vi "ConvertPrefStrings.vi"(6 "Comma?":bool, 8 "String In":string, 11 "Settings":T1={"Name of test"="", "Date"=timestamp(0 s since 1904-01-01), "Location"="Home", "Template"="Simple", "Soundcard"="OCTA-CAPTURE", "resolution"=32, "Sampling rate"=48000, "Ch1 Gain "=25.0, "Ch2 Gain"=10.0, "Sample time (s)"=0.3, "Pre-trigger (s)"=0.001, "Hammer Threshold"=10.0, "Positions"=12, "Taps/Position"=5, "Set Names"="H,V", "Freq resolution"=1.0, "Hammer cutoff"=0.025, "Mic cutoff"=0.25, "Double bounce "=10.0, "Hammer Cal"=10.0, "dB Offset"=0.0, "Accel Cal"=10.0, "Vibrometer Cal"=0.0, "Mic Cal"=0.0, "Output"=2, "Voltage Cal"=0.01, "Vibrometer Port"="ASRL27::INSTR", "Range"=4, "High Pass"=2, "Bandwidth"=4, "X Range"=[], "Y Range"=[], "dB Spread"=0.0, "Trigger"=0, "Ch_1"=25, "Ch_2"=25, "flip?"=FALSE, "60Hz"=FALSE, "Time offset"=0.0, "Piezo Cal"=1.0, "Default Notes"="", "Tom"=FALSE} {"Ch_2" min=1 step=1; "Ch_1" min=1 max=100 step=1; "Trigger" items=["Hammer (force)", "Self-tap", "Spacebar"]; "Bandwidth" items=["1 kHz"=1, "5 kHz"=5, "10 kHz"=10, "25 kHz"=25, "50 kHz"=50, "100 kHz"=100]; "High Pass" items=["Off", "13 Hz", "104 Hz"]; "Range" items=["10 mm/s"=1, "20 mm/s"=2, "50 mm/s"=5, "100 mm/s"=10, "200 mm/s"=20, "500 mm/s"=50, "1 m/s"=100, "2 m/s"=200]; "Output" items=["Accelerometer", "Speed (from acceleration)", "Microphone", "Vibrometer", "Piezo"]; "Voltage Cal" format="%#_13g"; "Ch2 Gain" format="%#_13g"; "Ch1 Gain" format="%#_13g"; "Double bounce" min=0.0; "Mic cutoff" min=0.0 format="%#_4g"; "Hammer cutoff" min=0.0 format="%#_4g"; "Freq resolution" min=0.0; "Pre-trigger (s)" format="%#_13g"; "Date" format="%<%H:%M\n%d/%m/%y>T"; "resolution" items=["16 bit"=16, "24 bit"=24, "32 bit"=32]; "Sampling rate" items=["22050 samp/s"=22050, "44100 samp/s"=44100, "48000 samp/s"=48000]}) -> (0 "Settings":T1={"Name of test"="", "Date"=timestamp(0 s since 1904-01-01), "Location"="", "Template"="", "Soundcard"="", "resolution"=32, "Sampling rate"=48000, "Ch1 Gain "=25.0, "Ch2 Gain"=10.0, "Sample time (s)"=0.3, "Pre-trigger (s)"=0.01, "Hammer Threshold"=10.0, "Positions"=12, "Taps/Position"=5, "Set Names"="", "Freq resolution"=10.0, "Hammer cutoff"=0.0, "Mic cutoff"=0.0, "Double bounce "=0.0, "Hammer Cal"=10.0, "dB Offset"=0.0, "Accel Cal"=10.0, "Vibrometer Cal"=0.0, "Mic Cal"=0.0, "Output"=2, "Voltage Cal"=0.01, "Vibrometer Port"="ASRL27::INSTR", "Range"=4, "High Pass"=2, "Bandwidth"=4, "X Range"=[], "Y Range"=[], "dB Spread"=0.0, "Trigger"=0, "Ch_1"=25, "Ch_2"=25, "flip?"=FALSE, "60Hz"=FALSE, "Time offset"=0.0, "Piezo Cal"=1.0, "Default Notes"="", "Tom"=FALSE} {"Ch_2" min=1 step=1; "Ch_1" min=1 max=100 step=1; "Trigger" items=["Hammer (force)", "Self-tap", "Spacebar"]; "Bandwidth" items=["1 kHz"=1, "5 kHz"=5, "10 kHz"=10, "25 kHz"=25, "50 kHz"=50, "100 kHz"=100]; "High Pass" items=["Off", "13 Hz", "104 Hz"]; "Range" items=["10 mm/s"=1, "20 mm/s"=2, "50 mm/s"=5, "100 mm/s"=10, "200 mm/s"=20, "500 mm/s"=50, "1 m/s"=100, "2 m/s"=200]; "Output" items=["Accelerometer", "Speed (from acceleration)", "Microphone", "Vibrometer", "Piezo"]; "Voltage Cal" format="%#_13g"; "Ch2 Gain" format="%#_13g"; "Ch1 Gain" format="%#_13g"; "Double bounce" min=0.0; "Mic cutoff" min=0.0 format="%#_4g"; "Hammer cutoff" min=0.0 format="%#_4g"; "Freq resolution" min=0.0; "Pre-trigger (s)" format="%#_13g"; "Date" format="%<%H:%M\n%d/%m/%y>T"; "resolution" items=["16 bit"=16, "24 bit"=24, "32 bit"=32]; "Sampling rate" items=["22050 samp/s"=22050, "44100 samp/s"=44100, "48000 samp/s"=48000]}, 3 "String Out":string)   [LabVIEW 2022 SP3]
uses:
  Mic/Mic_Global.vi
  PreferencesControl.ctl
panel:
  # "Hz"
  # "dB"
  # "dB"
  # "sec"
  # "sec"
  # "mV/Pa"
  # "mV/m/s2"
  # "mV/mm/s"
  # "V/N"
  # "sec"
  # "sec"
  # "mV/N"
  # "%"
  # "%"
  # "sec"
  # "Hz"
  # "dB"
  # "dB"
  # "sec"
  # "sec"
  # "mV/Pa"
  # "mV/m/s2"
  # "mV/mm/s"
  # "V/N"
  # "sec"
  # "sec"
  # "mV/N"
  # "%"
  # "%"
  # "sec"
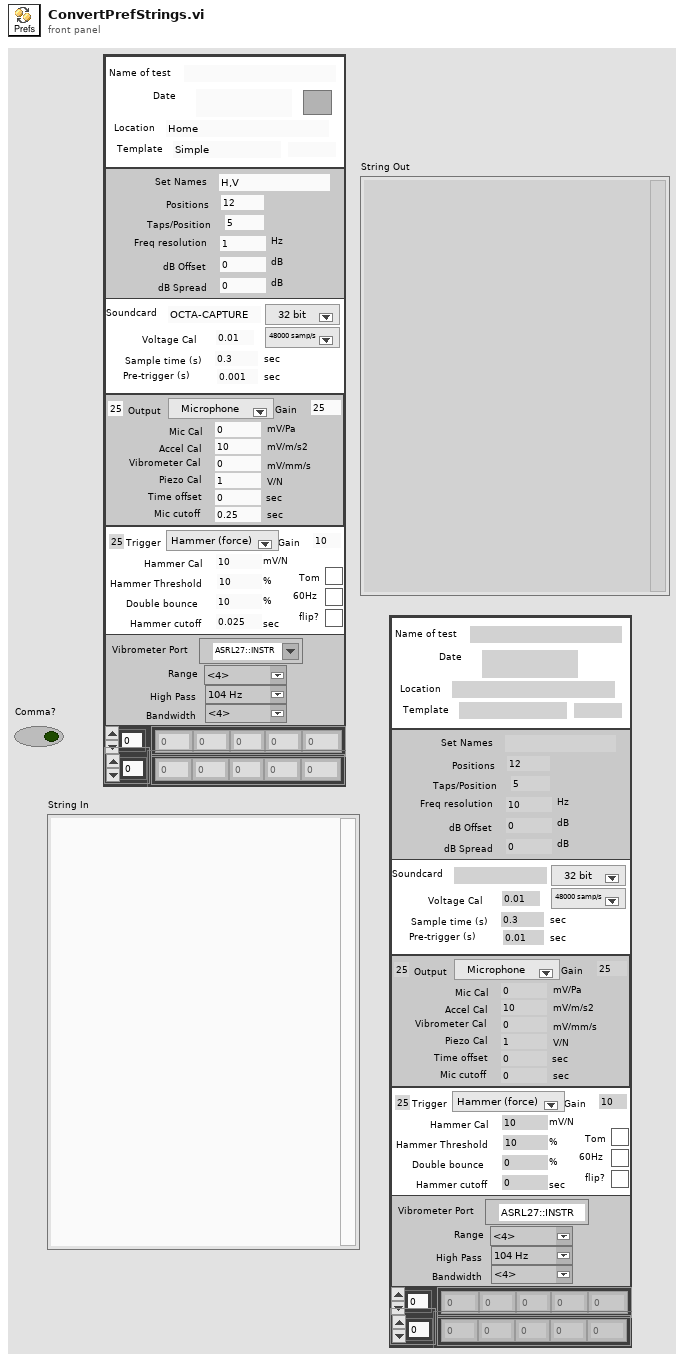
[diagram p1: front panel]
types:
  T1 = typedef "PreferencesControl.ctl" = cluster{"Name of test":string, "Date":timestamp, "Location":string, "Template":string, "Soundcard":string, "resolution":u16, "Sampling rate":u16, "Ch1 Gain ":dbl, "Ch2 Gain":dbl, "Sample time (s)":dbl, "Pre-trigger (s)":dbl, "Hammer Threshold":dbl, "Positions":i16, "Taps/Position":i16, "Set Names":string, "Freq resolution":dbl, "Hammer cutoff":dbl, "Mic cutoff":dbl, "Double bounce ":dbl, "Hammer Cal":dbl, "dB Offset":dbl, "Accel Cal":dbl, "Vibrometer Cal":dbl, "Mic Cal":dbl, "Output":u16, "Voltage Cal":dbl, "Vibrometer Port":refnum<visa-resource-name>, "Range":u16, "High Pass":u16, "Bandwidth":u16, "X Range":cluster{"Minimum":dbl, "Maximum":dbl, "Increment":dbl, "Minor Increment":dbl, "Start":dbl}[], "Y Range":cluster{"Minimum":dbl, "Maximum":dbl, "Increment":dbl, "Minor Increment":dbl, "Start":dbl}[], "dB Spread":dbl, "Trigger":u16, "Ch_1":u8, "Ch_2":u8, "flip?":bool, "60Hz":bool, "Time offset":dbl, "Piezo Cal":dbl, "Default Notes":string, "Tom":bool}
  T2 = typedef "LVStringsAndValuesArrayTypeDef_U16.ctl" = cluster{"String":string, "Value":u16}[]
  T3 = cluster{"Minimum":dbl, "Maximum":dbl, "Increment":dbl, "Minor Increment":dbl, "Start":dbl}[]
  T4 = cluster{"[0]":dbl, "[1]":dbl, "[2]":dbl, "[3]":dbl, "[4]":dbl}
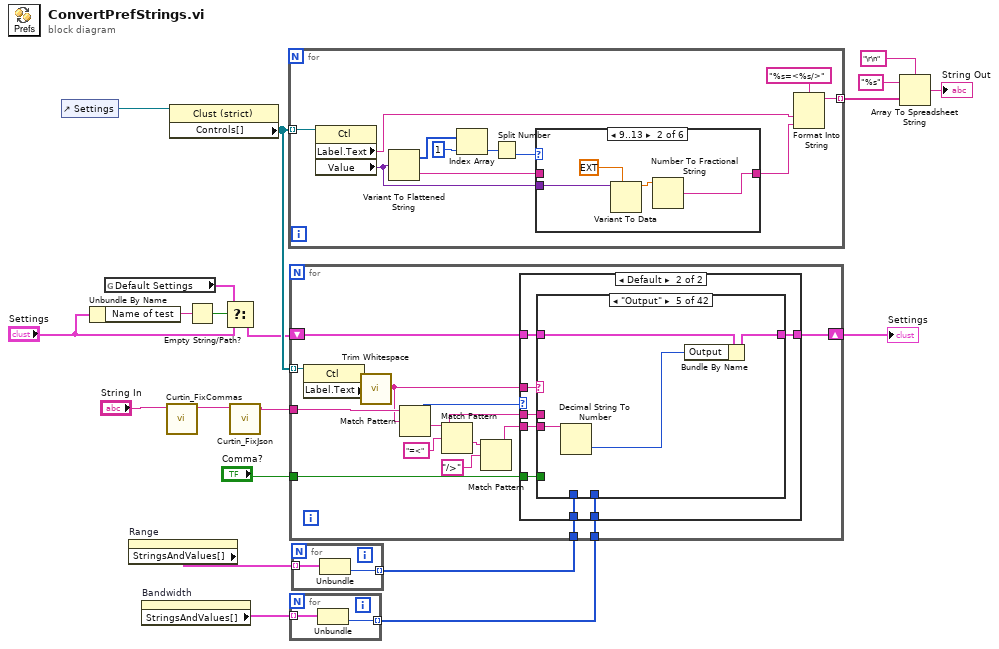
[diagram p0: block diagram]
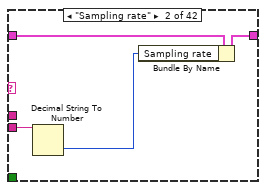
[diagram p4: hidden frame]
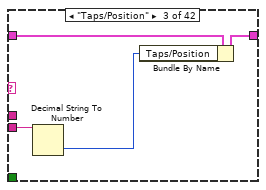
[diagram p5: hidden frame]
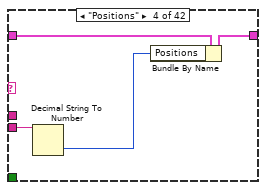
[diagram p6: hidden frame]
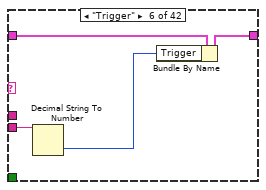
[diagram p7: hidden frame]
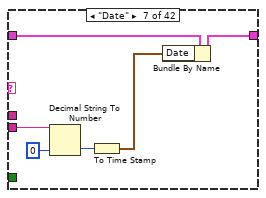
[diagram p8: hidden frame]
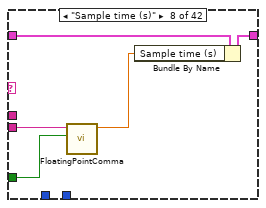
[diagram p9: hidden frame]
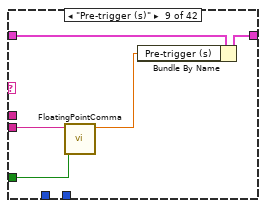
[diagram p10: hidden frame]
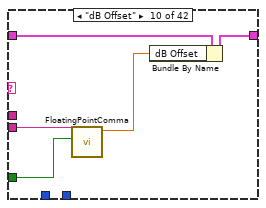
[diagram p11: hidden frame]
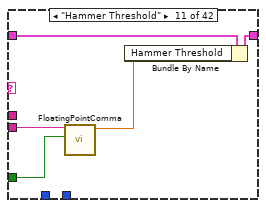
[diagram p12: hidden frame]
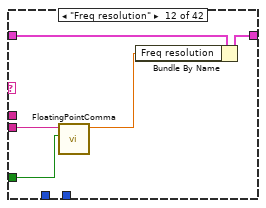
[diagram p13: hidden frame]
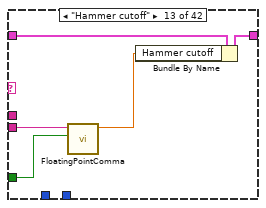
[diagram p14: hidden frame]
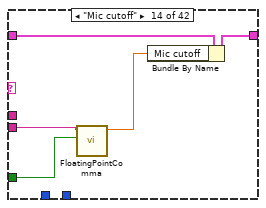
[diagram p15: hidden frame]
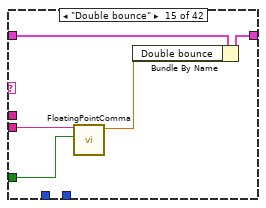
[diagram p16: hidden frame]
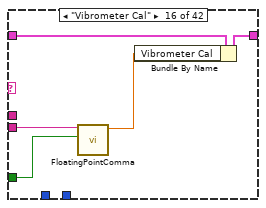
[diagram p17: hidden frame]
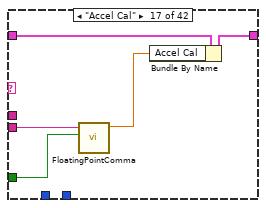
[diagram p18: hidden frame]
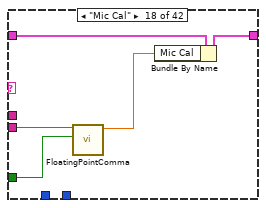
[diagram p19: hidden frame]
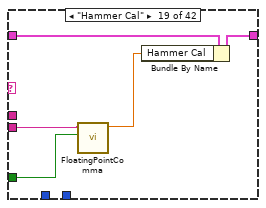
[diagram p20: hidden frame]
diagram:
  n1 = control-ref of="Settings"() -> (w14:refnum<vi>)
  n2 = Unbundle By Name("Settings") -> ("Name of test"=w13:string)
  n3 = global read "Mic_Global.vi" "Default Settings"() -> (w9:T1)
  n4 = property on="Range" class="Ring (strict)"() -> ("StringsAndValues[]"=w7:T2)  [unwired: 2 in, 2 out]
  n5 = property on="Bandwidth" class="Ring (strict)"() -> ("StringsAndValues[]"=w4:T2)  [unwired: 2 in, 2 out]
  n6 = call "Curtin_FixCommas.vi"("String In"="String In") -> ("String In 2"=w2:string)  [unwired: 10 in]
  n7 = property class="Clust (strict)"(reference=w14) -> ("Controls[]"=w16:refnum<vi>[])  [unwired: 1 in, 2 out]
  n8 = Empty String/Path?(string/path=w13) -> (empty?=w12:bool)
  n9 = Select(t=w9, s=w12, f="Settings") -> (s? t:f=w10:T1)
  n10 = call "Curtin_FixJson.vi"("String In"=w2) -> ("String out"=w1:string)  [unwired: 10 in]
  n11 = for {
    tunnel: w16 -> [w31] mode=indexing
    tunnel: [w29] -> w20 mode=indexing
    n12 = property class="Ctl"(reference=w31) -> ("Label.Text"=w22:string, "Value"=w23:variant)  [unwired: 1 in, 2 out]
    n13 = Variant To Flattened String(Variant=w23) -> (data string=w24:string, 1:w28:i16[])
    n14 = Index Array(array=w28, index=1) -> (element=w27:i16)
    n15 = Split Number(x=w27) -> (lo(x)=w21:u8)  [unwired: 1 out]
    n16 = case shown="9..13" w21 {
      tunnel: w23 -> [w35 w39 w45 w50 w56 _]
      tunnel: [w32 w36 w41 w46 w52 w63] -> w25
      tunnel: w24 -> [_ _ _ _ _ w66]
      frame 1..8 {
        n17 = Variant To Data(type=i64 0, Variant=w35) -> (data=w33:i64)  [unwired: 1 in, 1 out]
        n18 = Number To Decimal String(number=w33) -> (decimal integer string=w32:string)  [unwired: 1 in]
      }
      frame 9..13 {
        n19 = Variant To Data(type=ext 0.0, Variant=w39) -> (data=w37:ext)  [unwired: 1 in, 1 out]
        n20 = Number To Fractional String(number=w37) -> (F-format string=w36:string)  [unwired: 3 in]
      }
      frame 31, 33 {
        n21 = Variant To Data(type=FALSE, Variant=w45) -> (data=w43:bool)  [unwired: 1 in, 1 out]
        n22 = Select(t="true", s=w43, f="false") -> (s? t:f=w41:string)
      }
      frame 84 {
        n23 = Variant To Data(type=timestamp(0 s since 1904-01-01), Variant=w50) -> (data=w48:timestamp)  [unwired: 1 in, 1 out]
        n24 = To Unsigned Quad Integer(1:w48) -> (0:w47:u64)
        n25 = Number To Decimal String(number=w47) -> (decimal integer string=w46:string)  [unwired: 1 in]
      }
      frame 64 {
        n26 = Variant To Data(type=T3 [] ("X Range"), Variant=w56) -> (data=w54:T3)  [unwired: 1 in, 1 out]
        n27 = for {
          tunnel: w54 -> [w58] mode=indexing
          tunnel: [w57] -> w53 mode=indexing
          n28 = Cluster To Array(cluster=w58) -> (array=w57:dbl[])
        }
        n29 = Array To Spreadsheet String(array=w53, 3:"%e" ("format string")) -> (spreadsheet string=w52:string)  [unwired: 1 in]
      }
      frame 46, Default {
        n30 = Search/Split String(string=w66, offset (0)=4) -> (substring before match=w61:string, match + rest of string=w64:string)  [unwired: 1 in, 1 out]
        n31 = String To Byte Array(string=w61) -> (unsigned byte array=w60:u8[])
        n32 = Type Cast(type=4 ("offset (0)"), x=w60) -> ()  [unwired: 1 out]
        n33 = Format Into String(format string="%s", w64) -> (resulting string=w63:string)  [unwired: 2 in, 1 out]
      }
    }
    n34 = Format Into String(format string="%s=<%s/>", w22, w25) -> (resulting string=w29:string)  [unwired: 2 in, 1 out]
  }
  n35 = for {
    tunnel: w4 -> [w68] mode=indexing
    tunnel: [w67] -> w5 mode=indexing
    n36 = Unbundle(w68) -> ("Value"=w67:u16)  [unwired: 1 out]
  }
  n37 = for {
    tunnel: w7 -> [w70] mode=indexing
    tunnel: [w69] -> w6 mode=indexing
    n38 = Unbundle(w70) -> ("Value"=w69:u16)  [unwired: 1 out]
  }
  n39 = for {
    tunnel: w1 -> [w76]
    tunnel: w16 -> [w82] mode=indexing
    shift-right: [w80] -> w15
    shift-left: w10 -> [w81]
    tunnel: w6 -> [w73]
    tunnel: w5 -> [w72]
    tunnel: "Comma?" -> [w71]
    n40 = property class="Ctl"(reference=w82) -> ("Label.Text"=w75:string)  [unwired: 1 in, 2 out]
    n41 = call <vilib>:"Trim Whitespace.vi"("string"=w75) -> ("trimmed string"=w74:string)  [unwired: 1 in]
    n42 = Match Pattern(string=w76, regular expression=w74) -> (after substring=w77:string, offset past match=w78:i32)  [unwired: 1 in, 2 out]
    n43 = Match Pattern(string=w77, regular expression="=<" ("format string")) -> (after substring=w83:string)  [unwired: 1 in, 3 out]
    n44 = Match Pattern(string=w83, regular expression="/>" ("format string")) -> (before substring=w79:string)  [unwired: 1 in, 3 out]
    n45 = case shown="Default" w78 {
      tunnel: w81 -> [w86 w94]
      tunnel: [w86 w93] -> w80
      tunnel: w74 -> [_ w92]
      tunnel: w79 -> [_ w91]
      tunnel: w77 -> [_ w90]
      tunnel: w73 -> [_ w89]
      tunnel: w72 -> [_ w88]
      tunnel: w71 -> [_ w87]
      frame -1 {
      }
      frame Default {
        n46 = case shown="\"Output\"" w92 {
          tunnel: w94 -> [w95 w99 w103 w107 w111 w115 w121 w126 w131 w136 w141 w146 w151 w156 w161 w166 w171 w176 w181 w185 w188 w191 w194 w197 w200 w205 w210 w215 w218 w221 w230 w234 w243 w251 w261 w268 w272 w276 w281 w286 w291 w296]
          tunnel: [w95 w98 w102 w106 w110 w114 w120 w125 w130 w135 w140 w145 w150 w155 w160 w165 w170 w175 w180 w184 w187 w190 w193 w196 w199 w204 w209 w214 w217 w220 w229 w233 w242 w250 w260 w267 w271 w275 w280 w285 w290 w295] -> w93
          tunnel: w91 -> [_ w97 w101 w105 w109 w113 w119 w124 w129 w134 w139 w144 w149 w154 w159 w164 w169 w174 w179 w183 w186 w189 w192 w195 w198 w203 w208 w212 w216 w219 w223 w232 w241 w246 w256 w266 w270 w274 w278 w283 w288 w294]
          tunnel: w90 -> [_ _ _ _ _ _ _ _ _ _ _ _ _ _ _ _ _ _ _ _ _ _ _ _ _ _ _ _ _ _ _ _ _ _ _ _ _ _ _ _ _ _]
          tunnel: w89 -> [_ _ _ _ _ _ _ _ _ _ _ _ _ _ _ _ _ _ _ _ _ _ _ _ _ _ _ _ _ _ w222 _ _ _ _ _ _ _ _ _ _ _]
          tunnel: w88 -> [_ _ _ _ _ _ _ _ _ _ _ _ _ _ _ _ _ _ _ _ _ _ _ _ _ _ _ _ _ _ _ _ w237 _ _ _ _ _ _ _ _ _]
          tunnel: w87 -> [_ _ _ _ _ _ _ w122 w128 w133 w138 w143 w148 w153 w158 w163 w168 w173 w178 _ _ _ _ _ _ w202 w207 w213 _ _ _ _ _ w245 w255 w265 _ _ _ _ _ w293]
          frame Default {
          }
          frame "Sampling rate" {
            n47 = Decimal String To Number(string=w97) -> (number=w96:i32)  [unwired: 2 in, 1 out]
            n48 = Bundle By Name(cluster=w99, "Sampling rate"=w96) -> (w98:T1)
          }
          frame "Taps/Position" {
            n49 = Decimal String To Number(string=w101) -> (number=w100:i32)  [unwired: 2 in, 1 out]
            n50 = Bundle By Name(cluster=w103, "Taps/Position"=w100) -> (w102:T1)
          }
          frame "Positions" {
            n51 = Decimal String To Number(string=w105) -> (number=w104:i32)  [unwired: 2 in, 1 out]
            n52 = Bundle By Name(cluster=w107, "Positions"=w104) -> (w106:T1)
          }
          frame "Output" {
            n53 = Decimal String To Number(string=w109) -> (number=w108:i32)  [unwired: 2 in, 1 out]
            n54 = Bundle By Name(cluster=w111, "Output"=w108) -> (w110:T1)
          }
          frame "Trigger" {
            n55 = Decimal String To Number(string=w113) -> (number=w112:i32)  [unwired: 2 in, 1 out]
            n56 = Bundle By Name(cluster=w115, "Trigger"=w112) -> (w114:T1)
          }
          frame "Date" {
            n57 = Decimal String To Number(string=w119, default (0L)=u64 0 ("default (0 I32)")) -> (number=w118:u64)  [unwired: 1 in, 1 out]
            n58 = To Time Stamp(1:w118) -> (0:w117:timestamp)
            n59 = Bundle By Name(cluster=w121, "Date"=w117) -> (w120:T1)
          }
          frame "Sample time (s)" {
            n60 = call "FloatingPointComma.vi"("Comma?"=w122, "String In"=w124) -> ("Numeric"=w123:dbl)  [unwired: 8 in, 1 out]
            n61 = Bundle By Name(cluster=w126, "Sample time (s)"=w123) -> (w125:T1)
          }
          frame "Pre-trigger (s)" {
            n62 = call "FloatingPointComma.vi"("Comma?"=w128, "String In"=w129) -> ("Numeric"=w127:dbl)  [unwired: 8 in, 1 out]
            n63 = Bundle By Name(cluster=w131, "Pre-trigger (s)"=w127) -> (w130:T1)
          }
          frame "dB Offset" {
            n64 = call "FloatingPointComma.vi"("Comma?"=w133, "String In"=w134) -> ("Numeric"=w132:dbl)  [unwired: 8 in, 1 out]
            n65 = Bundle By Name(cluster=w136, "dB Offset"=w132) -> (w135:T1)
          }
          frame "Hammer Threshold" {
            n66 = call "FloatingPointComma.vi"("Comma?"=w138, "String In"=w139) -> ("Numeric"=w137:dbl)  [unwired: 8 in, 1 out]
            n67 = Bundle By Name(cluster=w141, "Hammer Threshold"=w137) -> (w140:T1)
          }
          frame "Freq resolution" {
            n68 = call "FloatingPointComma.vi"("Comma?"=w143, "String In"=w144) -> ("Numeric"=w142:dbl)  [unwired: 8 in, 1 out]
            n69 = Bundle By Name(cluster=w146, "Freq resolution"=w142) -> (w145:T1)
          }
          frame "Hammer cutoff" {
            n70 = call "FloatingPointComma.vi"("Comma?"=w148, "String In"=w149) -> ("Numeric"=w147:dbl)  [unwired: 8 in, 1 out]
            n71 = Bundle By Name(cluster=w151, "Hammer cutoff"=w147) -> (w150:T1)
          }
          frame "Mic cutoff" {
            n72 = call "FloatingPointComma.vi"("Comma?"=w153, "String In"=w154) -> ("Numeric"=w152:dbl)  [unwired: 8 in, 1 out]
            n73 = Bundle By Name(cluster=w156, "Mic cutoff"=w152) -> (w155:T1)
          }
          frame "Double bounce" {
            n74 = call "FloatingPointComma.vi"("Comma?"=w158, "String In"=w159) -> ("Numeric"=w157:dbl)  [unwired: 8 in, 1 out]
            n75 = Bundle By Name(cluster=w161, "Double bounce"=w157) -> (w160:T1)
          }
          frame "Vibrometer Cal" {
            n76 = call "FloatingPointComma.vi"("Comma?"=w163, "String In"=w164) -> ("Numeric"=w162:dbl)  [unwired: 8 in, 1 out]
            n77 = Bundle By Name(cluster=w166, "Vibrometer Cal"=w162) -> (w165:T1)
          }
          frame "Accel Cal" {
            n78 = call "FloatingPointComma.vi"("Comma?"=w168, "String In"=w169) -> ("Numeric"=w167:dbl)  [unwired: 8 in, 1 out]
            n79 = Bundle By Name(cluster=w171, "Accel Cal"=w167) -> (w170:T1)
          }
          frame "Mic Cal" {
            n80 = call "FloatingPointComma.vi"("Comma?"=w173, "String In"=w174) -> ("Numeric"=w172:dbl)  [unwired: 8 in, 1 out]
            n81 = Bundle By Name(cluster=w176, "Mic Cal"=w172) -> (w175:T1)
          }
          frame "Hammer Cal" {
            n82 = call "FloatingPointComma.vi"("Comma?"=w178, "String In"=w179) -> ("Numeric"=w177:dbl)  [unwired: 8 in, 1 out]
            n83 = Bundle By Name(cluster=w181, "Hammer Cal"=w177) -> (w180:T1)
          }
          frame "resolution" {
            n84 = Decimal String To Number(string=w183) -> (number=w182:i32)  [unwired: 2 in, 1 out]
            n85 = Bundle By Name(cluster=w185, "resolution"=w182) -> (w184:T1)
          }
          frame "Soundcard" {
            n86 = Bundle By Name(cluster=w188, "Soundcard"=w186) -> (w187:T1)
          }
          frame "Name of test" {
            n87 = Bundle By Name(cluster=w191, "Name of test"=w189) -> (w190:T1)
          }
          frame "Set Names" {
            n88 = Bundle By Name(cluster=w194, "Set Names"=w192) -> (w193:T1)
          }
          frame "Location" {
            n89 = Bundle By Name(cluster=w197, "Location"=w195) -> (w196:T1)
          }
          frame "Default Template" {
            n90 = Bundle By Name(cluster=w200, "Template"=w198) -> (w199:T1)
          }
          frame "Ch1 Gain" {
            n91 = call "FloatingPointComma.vi"("Comma?"=w202, "String In"=w203) -> ("Numeric"=w201:dbl)  [unwired: 8 in, 1 out]
            n92 = Bundle By Name(cluster=w205, "Ch1 Gain"=w201) -> (w204:T1)
          }
          frame "Ch2 Gain" {
            n93 = call "FloatingPointComma.vi"("Comma?"=w207, "String In"=w208) -> ("Numeric"=w206:dbl)  [unwired: 8 in, 1 out]
            n94 = Bundle By Name(cluster=w210, "Ch2 Gain"=w206) -> (w209:T1)
          }
          frame "Voltage Cal" {
            n95 = call "FloatingPointComma.vi"("Comma?"=w213, "String In"=w212) -> ("Numeric"=w211:dbl)  [unwired: 8 in, 1 out]
            n96 = Bundle By Name(cluster=w215, "Voltage Cal"=w211) -> (w214:T1)
          }
          frame "Vibrometer Port" {
            n97 = Bundle By Name(cluster=w218, "Vibrometer Port"=w216) -> (w217:T1)
          }
          frame "Default Notes" {
            n98 = Bundle By Name(cluster=w221, "Default Notes"=w219) -> (w220:T1)
          }
          frame "Range" {
            n99 = Decimal String To Number(string=w223) -> (number=w226:i32)  [unwired: 2 in, 1 out]
            n100 = Search 1D Array(1D array=w222, element=w226) -> (index of element=w228:i32)  [unwired: 1 in]
            n101 = Greater Or Equal To 0?(x=w228) -> (x >= 0?=w227:bool)
            n102 = Select(t=w226, s=w227, f=20) -> (s? t:f=w225:i32)
            n103 = Bundle By Name(cluster=w230, "Range"=w225) -> (w229:T1)
          }
          frame "High Pass" {
            n104 = Decimal String To Number(string=w232) -> (number=w231:i32)  [unwired: 2 in, 1 out]
            n105 = Bundle By Name(cluster=w234, "High Pass"=w231) -> (w233:T1)
          }
          frame "Bandwidth" {
            n106 = Decimal String To Number(string=w241) -> (number=w236:i32)  [unwired: 2 in, 1 out]
            n107 = Search 1D Array(1D array=w237, element=w236) -> (index of element=w240:i32)  [unwired: 1 in]
            n108 = Greater Or Equal To 0?(x=w240) -> (x >= 0?=w239:bool)
            n109 = Select(t=w236, s=w239, f=25) -> (s? t:f=w235:i32)
            n110 = Bundle By Name(cluster=w243, "Bandwidth"=w235) -> (w242:T1)
          }
          frame "X Range" {
            n111 = call "FloatingPointComma.vi"("Comma?"=w245, "String In"=w246) -> ("fixed"=w244:string)  [unwired: 8 in, 1 out]
            n112 = Spreadsheet String To Array(format string="%e", spreadsheet string=w244) -> (array=w248:dbl[][])  [unwired: 2 in]
            n113 = for {
              tunnel: w248 -> [w253] mode=indexing
              tunnel: [w252] -> w247 mode=indexing
              n114 = Array To Cluster(array=w253) -> (cluster=w252:T4)
            }
            n115 = Bundle By Name(cluster=w251, "X Range"=w247) -> (w250:T1)
          }
          frame "Y Range" {
            n116 = call "FloatingPointComma.vi"("Comma?"=w255, "String In"=w256) -> ("fixed"=w254:string)  [unwired: 8 in, 1 out]
            n117 = Spreadsheet String To Array(format string="%e", spreadsheet string=w254) -> (array=w258:dbl[][])  [unwired: 2 in]
            n118 = for {
              tunnel: w258 -> [w263] mode=indexing
              tunnel: [w262] -> w257 mode=indexing
              n119 = Array To Cluster(array=w263) -> (cluster=w262:T4)
            }
            n120 = Bundle By Name(cluster=w261, "Y Range"=w257) -> (w260:T1)
          }
          frame "dB Spread" {
            n121 = call "FloatingPointComma.vi"("Comma?"=w265, "String In"=w266) -> ("Numeric"=w264:dbl)  [unwired: 8 in, 1 out]
            n122 = Bundle By Name(cluster=w268, "dB Spread"=w264) -> (w267:T1)
          }
          frame "Ch_1" {
            n123 = Decimal String To Number(string=w270) -> (number=w269:i32)  [unwired: 2 in, 1 out]
            n124 = Bundle By Name(cluster=w272, "Ch_1"=w269) -> (w271:T1)
          }
          frame "Ch_2" {
            n125 = Decimal String To Number(string=w274) -> (number=w273:i32)  [unwired: 2 in, 1 out]
            n126 = Bundle By Name(cluster=w276, "Ch_2"=w273) -> (w275:T1)
          }
          frame "flip?" {
            n127 = Equal?(x="true", y=w278) -> (x = y?=w277:bool)
            n128 = Bundle By Name(cluster=w281, "flip?"=w277) -> (w280:T1)
          }
          frame "60Hz" {
            n129 = Equal?(x="true", y=w283) -> (x = y?=w282:bool)
            n130 = Bundle By Name(cluster=w286, "60Hz"=w282) -> (w285:T1)
          }
          frame "Tom" {
            n131 = Equal?(x="true", y=w288) -> (x = y?=w287:bool)
            n132 = Bundle By Name(cluster=w291, "Tom"=w287) -> (w290:T1)
          }
          frame "Time offset" {
            n133 = call "FloatingPointComma.vi"("Comma?"=w293, "String In"=w294) -> ("Numeric"=w292:dbl)  [unwired: 8 in, 1 out]
            n134 = Bundle By Name(cluster=w296, "Time offset"=w292) -> (w295:T1)
          }
        }
      }
    }
  }
  "Settings" <- w15
  n135 = Array To Spreadsheet String(delimiter (Tab)="\r\n", array=w20, 3:"%s" ("format string")) -> (spreadsheet string=→"String Out":string)
